vi "Write FXP.vi"(7 "FXP Configuration":T1, 8 "error in":errorcluster, 9 "DBL Value":dbl, 10 "register offset":u32, 11 "session in":u32) -> (0 "error out":errorcluster, 3 "session out":u32)   [LabVIEW 2018, in "Scalar IO Operations.lvlib"]
uses:
  Scalar IO Operations.lvlib
  TypeDefs/FXP Configuration.ctl
  <vilib>/fxp/LVFixedPointRepBitsTypeDef.ctl
  <vilib>/fxp/LVFixedPointRepRangeTypeDef.ctl
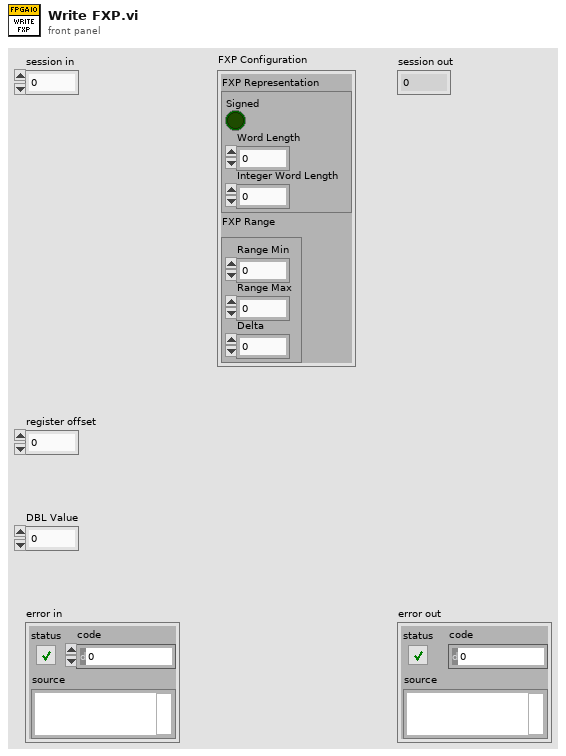
[diagram p1: front panel]
types:
  T1 = typedef "Scalar IO Operations.lvlib/FXP Configuration.ctl" = cluster{"FXP Representation":T2, "FXP Range":T3}
  T2 = typedef "LVFixedPointRepBitsTypeDef.ctl" = cluster{"Signed":bool, "Word Length":u32, "Integer Word Length":i32}
  T3 = typedef "LVFixedPointRepRangeTypeDef.ctl" = cluster{"Range Min":dbl, "Range Max":dbl, "Delta":dbl}
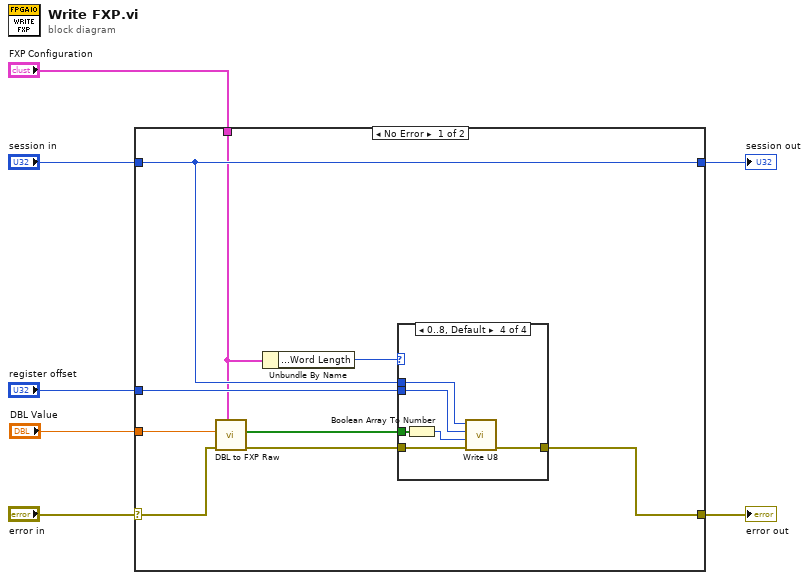
[diagram p0: block diagram]
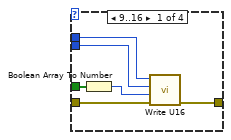
[diagram p2: hidden frame]
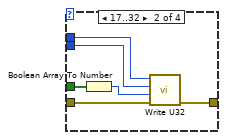
[diagram p3: hidden frame]
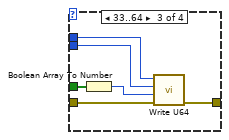
[diagram p4: hidden frame]
diagram:
  n1 = case shown="No Error" "error in" {
    selector: "error in" -> [w13 w42]
    tunnel: "session in" -> [w15 w41]
    tunnel: [w14 w42] -> w6
    tunnel: "register offset" -> [w16 _]
    tunnel: [w15 w41] -> w3
    tunnel: "FXP Configuration" -> [w8 _]
    tunnel: "DBL Value" -> [w11 _]
    frame No Error {
      n2 = call "DBL to FXP Raw.vi"("FXP Configuration"=w8, "error in (no error)"=w13, "DBL Value"=w11) -> ("error out"=w12:errorcluster, "Bool Data"=w10:bool[])  [unwired: 7 in]
      n3 = Unbundle By Name(w8) -> ("FXP Representation.Word Length"=w9:u32)
      n4 = case shown="0..8, Default" w9 {
        tunnel: w16 -> [w19 w25 w31 w38]
        tunnel: w15 -> [w20 w26 w30 w39]
        tunnel: w12 -> [w22 w28 w34 w40]
        tunnel: [w21 w27 w33 w37] -> w14
        tunnel: w10 -> [w18 w24 w32 w36]
        frame 9..16 {
          n5 = Boolean Array To Number(Boolean array=w18) -> (number=w17:u16)
          n6 = call "Write U16.vi"("error in"=w22, "value in"=w17, "register offset"=w19, "session in"=w20) -> ("error out"=w21:errorcluster)  [unwired: 6 in, 1 out]
        }
        frame 17..32 {
          n7 = Boolean Array To Number(Boolean array=w24) -> (number=w23:u32)
          n8 = call "Write U32.vi"("error in"=w28, "value in"=w23, "register offset"=w25, "session in"=w26) -> ("error out"=w27:errorcluster)  [unwired: 6 in, 1 out]
        }
        frame 33..64 {
          n9 = Boolean Array To Number(Boolean array=w32) -> (number=w29:u64)
          n10 = call "Write U64.vi"("error in"=w34, "value in"=w29, "register offset"=w31, "session in"=w30) -> ("error out"=w33:errorcluster)  [unwired: 6 in, 1 out]
        }
        frame 0..8, Default {
          n11 = Boolean Array To Number(Boolean array=w36) -> (number=w35:u8)
          n12 = call "Write U8.vi"("error in"=w40, "value in"=w35, "register offset"=w38, "session in"=w39) -> ("error out"=w37:errorcluster)  [unwired: 6 in, 1 out]
        }
      }
    }
    frame Error {
    }
  }
  "error out" <- w6
  "session out" <- w3
